vi "(SubVI)I2C_Run Macro.vi"(5 "Log Ref":refnum<vi>, 8 "error in (no error)":errorcluster caption="에러 입력(에러 없음)", 11 "Macro File Path in":path) -> (0 "error out":errorcluster caption="에러 출력", 3 "Macro File Path Out":path)   [LabVIEW 2020]
uses:
  Instance VIs/(SubVI)I2C_16Bit-16Bit_Read_Single.vi
  Instance VIs/(SubVI)I2C_16Bit-16Bit_Write_Single.vi
panel:
  # "(SubVI)I2C_Run Macro.vi By hspark\n\nDescription : I2C Macro File을 읽어서 Read/Write를 실행하는 VI\n\nInput : \n1. Macro File Path In : 매크로 파일 경로 입력\n2. Log Ref : Macro File 실행 결과를 Log에 남기기 위해 Log 문자열 인디케이터의 참조를 입력.\n                참조를 입력하지 않으면 인디케이터에 Log를 남기지 않음.\n\nOutput : \n1. Macro File Path Out : 매크로파일 경로 출력\n\nLabVIEW Version : 2020 SP1 이상\n\nNote : \n기존 OISLab과 동일한 양식의 Macro File을 사용하도록 작성하였음. \n단, Delay 뒤에 숫자 값을 입력하여 Delay 지정이 가능함. (숫자 값 없이 Delay 사용 시 10ms)\n\nUpdate : 2021.10.06"
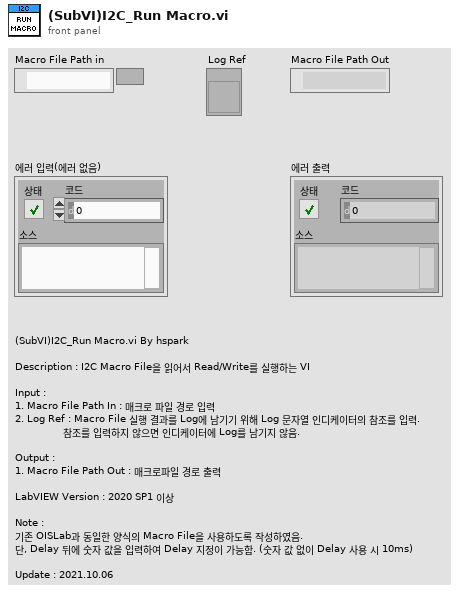
[diagram p1: front panel]
types:
  T1 = cluster{"Type":enum16{"I2C Read", "I2C Write", "Delay"}, "ID":u8, "Address":u16, "Data":u16, "Delay(ms)":u32}
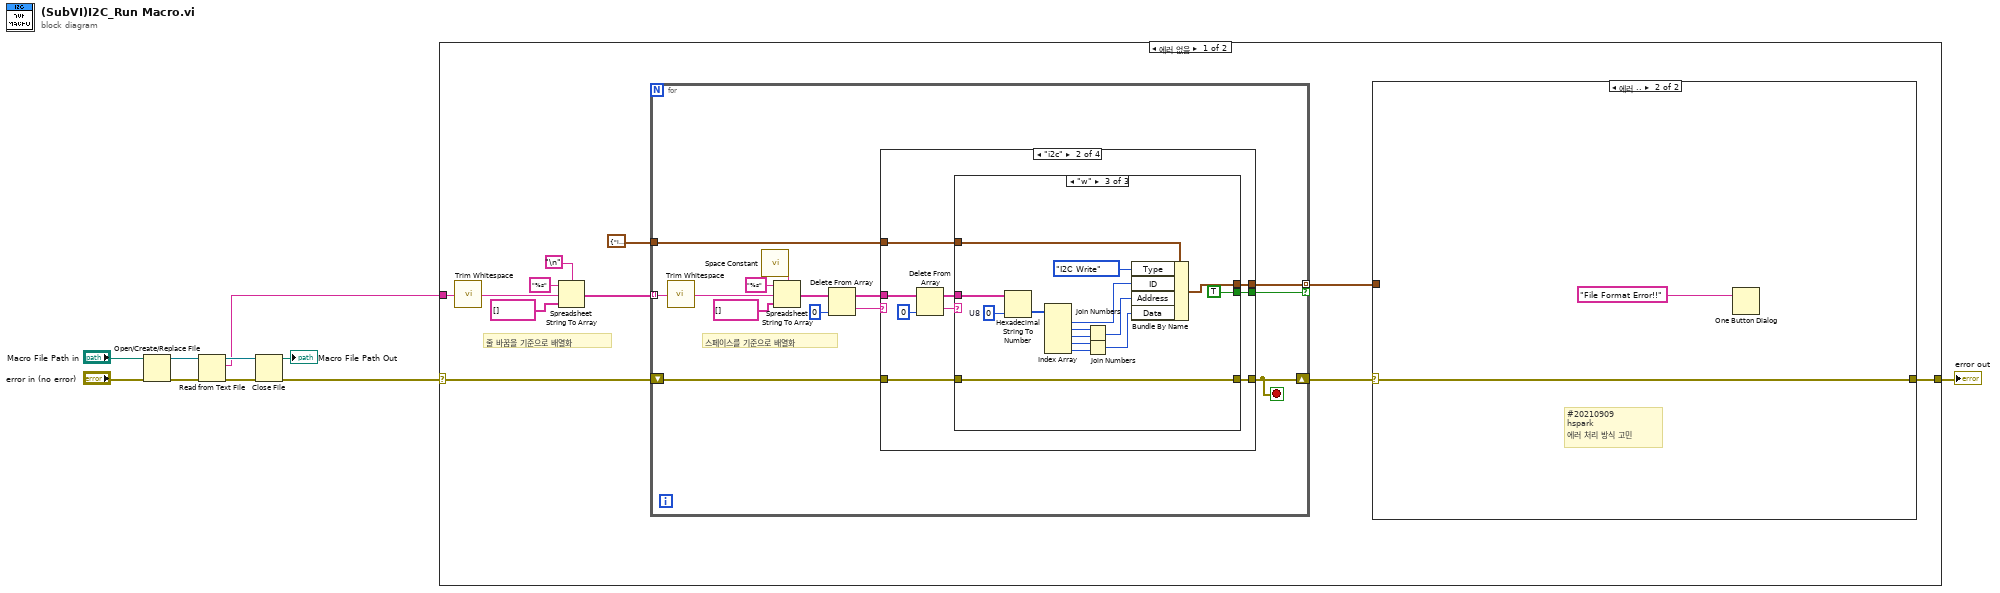
[diagram p0: block diagram]
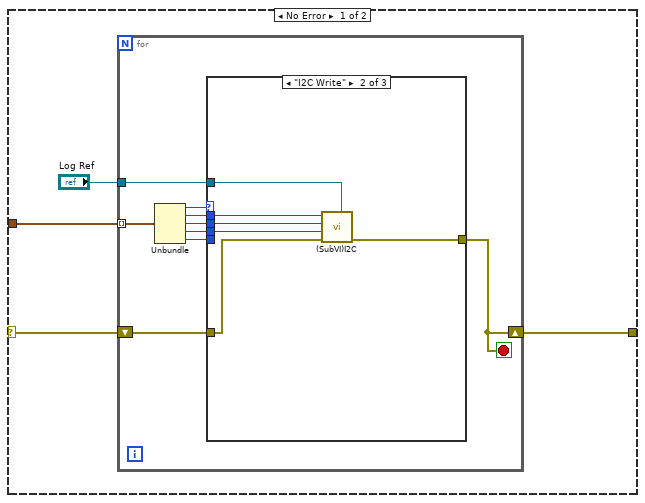
[diagram p2: hidden frame]
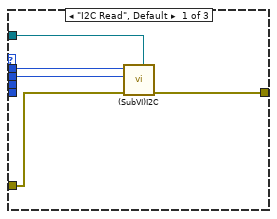
[diagram p3: hidden frame]
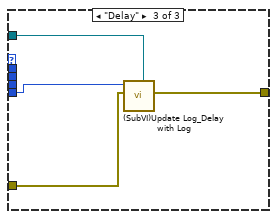
[diagram p4: hidden frame]
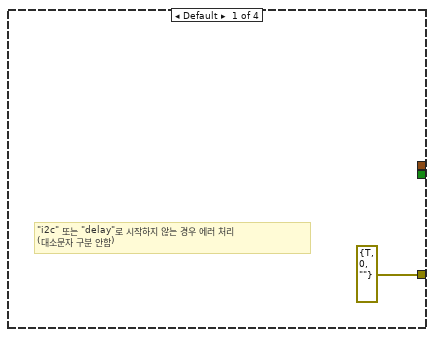
[diagram p5: hidden frame]
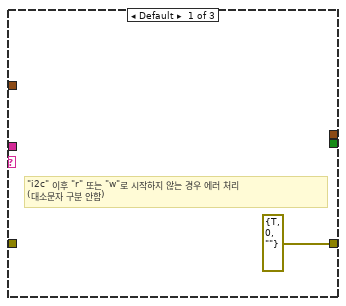
[diagram p6: hidden frame]
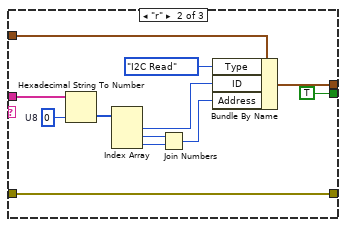
[diagram p7: hidden frame]
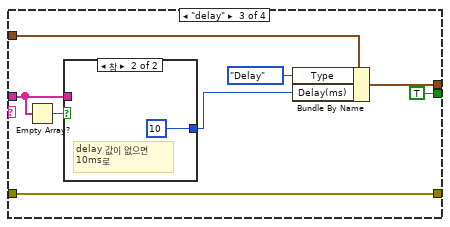
[diagram p8: hidden frame]
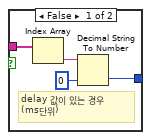
[diagram p9: hidden frame]
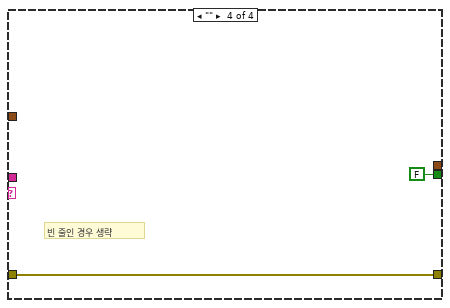
[diagram p10: hidden frame]
diagram:
  n1 = Open/Create/Replace File(file path (use dialog)="Macro File Path in", error in="error in (no error)") -> (refnum out=w8:refnum<file>, error out=w7:errorcluster)  [unwired: 4 in, 1 out]
  n2 = Read from Text File(file (use dialog)=w8, error in=w7) -> (refnum out=w6:refnum<file>, text=w4:string, error out=w5:errorcluster)  [unwired: 2 in, 1 out]
  n3 = Close File(refnum=w6, error in=w5) -> (path=→"Macro File Path Out":path, error out=w3:errorcluster)
  n4 = case shown="에러 없음" w3 {
    selector: w3 -> [w13 w119]
    tunnel: w4 -> [w14 _]
    tunnel: [w11 w119] -> w2
    frame No Error {
      # "줄 바꿈을 기준으로 배열화"
      n5 = call <vilib>:"Trim Whitespace.vi"("string"=w14) -> ("trimmed string"=w16:string)  [unwired: 1 in]
      n6 = Spreadsheet String To Array(delimiter (Tab)="\n", format string="%s" ("포맷 문자열"), spreadsheet string=w16, array type (2D Dbl)=string[] []) -> (array=w18:string[])
      n7 = for {
        tunnel: w18 -> [w65] mode=indexing
        tunnel: T1 {"Type"=enum."I2C Read", "ID"=0, "Address"=0, "Data"=0, "Delay(ms)"=0} -> [w57]
        tunnel: [w56] -> w15 mode=indexing if=w52
        shift-right: [w54] -> w12
        shift-left: w13 -> [w55]
        stop <- w54 stop-if-true
        # "스페이스를 기준으로 배열화"
        n8 = call <vilib>:"Trim Whitespace.vi"("string"=w65) -> ("trimmed string"=w53:string)  [unwired: 1 in]
        n9 = call <vilib>:"Space Constant.vi"() -> ("String"=w63:string)
        n10 = Spreadsheet String To Array(delimiter (Tab)=w63, format string="%s" ("포맷 문자열"), spreadsheet string=w53, array type (2D Dbl)=string[] []) -> (array=w61:string[])
        n11 = Delete From Array(array=w61, index=0 ("인덱스")) -> (deleted portion=w59:string, array with subset deleted=w58:string[])  [unwired: 1 in]
        n12 = case shown="\"i2c\"" w59 {
          tunnel: w58 -> [_ w74 w108 _]
          tunnel: w57 -> [_ w71 w111 _]
          tunnel: [_ w70 w110 _] -> w56
          tunnel: w55 -> [_ w69 w105 w118]
          tunnel: [errorcluster {"status"=TRUE, "code"=0, "source"=""} ("error IO") w68 w105 w118] -> w54
          tunnel: [_ w67 TRUE FALSE] -> w52
          frame Default {
            # "\"i2c\" 또는 \"delay\"로 시작하지 않는 경우 에러 처리\n(대소문자 구분 안함)"
          }
          frame "i2c" {
            n13 = Delete From Array(array=w74, index=0 ("인덱스")) -> (deleted portion=w73:string, array with subset deleted=w72:string[])  [unwired: 1 in]
            n14 = case shown="\"w\"" w73 {
              tunnel: w72 -> [_ w86 w101]
              tunnel: w71 -> [_ w88 w103]
              tunnel: [_ w79 w91] -> w70
              tunnel: w69 -> [_ w78 w90]
              tunnel: [errorcluster {"status"=TRUE, "code"=0, "source"=""} ("error out") w78 w90] -> w68
              tunnel: [_ TRUE TRUE] -> w67
              frame Default {
                # "\"i2c\" 이후 \"r\" 또는 \"w\"로 시작하지 않는 경우 에러 처리\n(대소문자 구분 안함)"
              }
              frame "r" {
                w85 = u8 0  # U8
                n15 = Hexadecimal String To Number(string=w86, default (0uL)=w85) -> (number=w84:u8[])  [unwired: 1 in, 1 out]
                n16 = Index Array(array=w84) -> (element #1=w81:u8, element #2=w83:u8, element #3=w82:u8)  [unwired: 3 in]
                n17 = Join Numbers(hi=w83, lo=w82) -> ((hi.lo)=w80:u16)
                n18 = Bundle By Name(cluster=w88, "Type"=enum16{"I2C Read", "I2C Write", "Delay"}."I2C Read", "ID"=w81, "Address"=w80) -> (w79:T1)
              }
              frame "w" {
                w100 = u8 0  # U8
                n19 = Hexadecimal String To Number(string=w101, default (0uL)=w100) -> (number=w99:u8[])  [unwired: 1 in, 1 out]
                n20 = Index Array(array=w99) -> (element #1=w97:u8, element #2=w98:u8, element #3=w95:u8, element #4=w94:u8, element #5=w93:u8)  [unwired: 5 in]
                n21 = Join Numbers(hi=w98, lo=w95) -> ((hi.lo)=w96:u16)
                n22 = Join Numbers(hi=w94, lo=w93) -> ((hi.lo)=w92:u16)
                n23 = Bundle By Name(cluster=w103, "Type"=enum16{"I2C Read", "I2C Write", "Delay"}."I2C Write", "ID"=w97, "Address"=w96, "Data"=w92) -> (w91:T1)
              }
            }
          }
          frame "delay" {
            n24 = Empty Array?(array=w108) -> (empty?=w107:bool)
            n25 = case shown="참" w107 {
              tunnel: w108 -> [w115 _]
              tunnel: [w113 u32 10 ("Delay")] -> w106
              frame False {
                # "delay 값이 있는 경우\n(ms단위)"
                n26 = Index Array(array=w115) -> (element=w114:string)  [unwired: 1 in]
                n27 = Decimal String To Number(string=w114, default (0L)=u32 0 ("기본(0 I32)")) -> (number=w113:u32)  [unwired: 1 in, 1 out]
              }
              frame True {
                # "delay 값이 없으면\n10ms로"
              }
            }
            n28 = Bundle By Name(cluster=w111, "Type"=enum16{"I2C Read", "I2C Write", "Delay"}."Delay", "Delay(ms)"=w106) -> (w110:T1)
          }
          frame "" {
            # "빈 줄인 경우 생략"
          }
        }
      }
      n29 = case shown="에러 .." w12 {
        selector: w12 -> [w24 w50]
        tunnel: w15 -> [w25 _]
        tunnel: [w23 w50] -> w11
        frame No Error {
          n30 = for {
            tunnel: w25 -> [w34] mode=indexing
            shift-right: [w27] -> w23
            shift-left: w24 -> [w28]
            tunnel: "Log Ref" -> [w26]
            stop <- w27 stop-if-true
            n31 = Unbundle(w34) -> ("Type"=w33:enum16{"I2C Read", "I2C Write", "Delay"}, "ID"=w32:u8, "Address"=w31:u16, "Data"=w30:u16, "Delay(ms)"=w29:u32)
            n32 = case shown="\"I2C Write\"" w33 {
              tunnel: w32 -> [w39 w45 _]
              tunnel: w31 -> [w38 w44 _]
              tunnel: w30 -> [_ w43 _]
              tunnel: w29 -> [_ _ w49]
              tunnel: w28 -> [w37 w42 w48]
              tunnel: [w36 w41 w47] -> w27
              tunnel: w26 -> [w35 w40 w46]
              frame "I2C Read", Default {
                n33 = call-poly "(SubVI)I2C.vi"("Log Ref"=w35, "error in (no error)"=w37, "Address"=w38, "ID"=w39) -> ("error out"=w36:errorcluster)  [unwired: 5 in, 2 out]
              }
              frame "I2C Write" {
                n34 = call-poly "(SubVI)I2C.vi"("Log Ref"=w40, "error in (no error)"=w42, "Data to Write"=w43, "Address"=w44, "ID"=w45) -> ("error out"=w41:errorcluster)  [unwired: 5 in, 1 out]
              }
              frame "Delay" {
                n35 = call "(SubVI)Update Log_Delay with Log.vi"("Log Ref"=w46, "error in (no error)"=w48, "Delay (ms)"=w49) -> ("error out"=w47:errorcluster)  [unwired: 7 in, 1 out]
              }
            }
          }
        }
        frame Error {
          # "#20210909\nhspark\n에러 처리 방식 고민"
          n36 = One Button Dialog(message="File Format Error!!" ("메시지")) -> ()  [unwired: 1 in, 1 out]
        }
      }
    }
    frame Error {
    }
  }
  "error out" <- w2
